vi "FPGA-Top-Level.vi"() -> ()   [LabVIEW 2015]
uses:
  <vilib>/rvi/DataTransferAndStorage/Container/Common/niFpgaContainerExecOnDevCompGetState.vi
  <vilib>/rvi/Emulation/niFpgaEmulationIsFPGAContextNoSignature.vi
  <vilib>/rvi/DataTransferAndStorage/Container/Common/niFpgaContainerGetUniqueNameForEmu.vi
  <vilib>/rvi/Emulation/niFpgaProcessEmulError.vi
  <vilib>/rvi/Emulation/niFpgaSctlEmulationGetInTimedLoop.vi
  <vilib>/rvi/errors/nirviReportUnexpectedCaseInternalError (U32).vi
  <vilib>/rvi/Memory/Memory_Emulation/niFpgaMemoryEmulationCacheClearOnFirstRun.vi
  <vilib>/rvi/Memory/Memory_Emulation/nirvimemoryEmulationManagerCache_MakeExclusive.vi
  <vilib>/rvi/Memory/Memory_Emulation/niFpgaMemoryEmulationValidateCache.vi
  <vilib>/rvi/Memory/Memory_Emulation/nirvimemoryEmulationManagerCache_InsertValue.vi
  <vilib>/Utility/error.llb/Clear Errors.vi
  <vilib>/rvi/Memory/Memory_Emulation/nirvimemoryEmulationManagerCache_ReleaseExclusive.vi
  <vilib>/rvi/Memory/Memory_Emulation/nirvimemoryEmulationManagerCache_GetValue.vi
  <vilib>/rvi/Memory/Memory_Emulation/nirvimemoryEmulationManagerCache_SetValue.vi
  <vilib>/rvi/Emulation/niFpgaSctlEmulationResourceMgr.vi
  <vilib>/rvi/DataTransferAndStorage/Container/Common/niFpgaContainerSetEmuInfo.vi
  <vilib>/rvi/eio/common/nirviEmuReportErrorAndStop.vi
  <vilib>/rvi/DataTransferAndStorage/Container/XNode/niFpgaContainer.xnode
  <vilib>/rvi/Memory/Memory_Emulation/niFpgaMemoryEmulationRefIn.vi
  <vilib>/rvi/LocalResourceManager/LocalResourceManager.xnode
panel:
  out "FPGA-Global":u64
  out "VI_Defined":u64
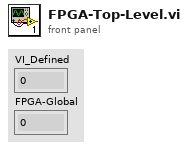
[diagram p1: front panel]
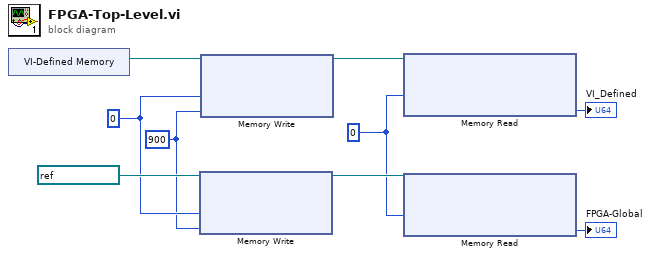
[diagram p0: block diagram]
diagram:
  w3 = u32 0 ("Address")
  w6 = u64 900 ("Data")
  w7 = u32 0 ("Address")
  n1 = xnode "VI-Defined Memory"() -> ("Memory Out"=w9:refnum<k21>)
  n2 = xnode "Memory Write"("Address"=w7, "Data"=w6, "Memory In"=refnum<k21> "My_SRAM") -> ("Memory Out"=w5:refnum<k21>)
  n3 = xnode "Memory Write"("Address"=w7, "Data"=w6, "Memory In"=w9) -> ("Memory Out"=w4:refnum<k21>)
  n4 = xnode "Memory Read"("Address"=w3, "Memory In"=w4) -> ("Data"=→"VI_Defined":u64)  [unwired: 1 out]
  n5 = xnode "Memory Read"("Address"=w3, "Memory In"=w5) -> ("Data"=→"FPGA-Global":u64)  [unwired: 1 out]
